vi "Test Error Test.vi"(8 "error in (no error)":errorcluster, 11 "LUnit Test Case V2 Test Double in":refnum<class "LUnit Test Case V2 Test Double.lvclass">) -> (0 "error out":errorcluster, 3 "LUnit Test Case V2 Test Double out":refnum<class "LUnit Test Case V2 Test Double.lvclass">)   [LabVIEW 2020, in "LUnit Test Case V2 Test Double.lvclass"]
uses:
  LUnit Test Case V2 Test Double.lvclass
  C:/Git/astemes-lunit/source/Rewrite Project/LUnit Test Case/LUnit Test Case V2.lvclass
  LUnit Test Case/LUnit Test Case V2.lvclass/LUnit Test Case V2.ctl
  LUnit Test Case/Private/Append Result.vi
  LUnit Test Case/LUnit Test Case V2.lvclass
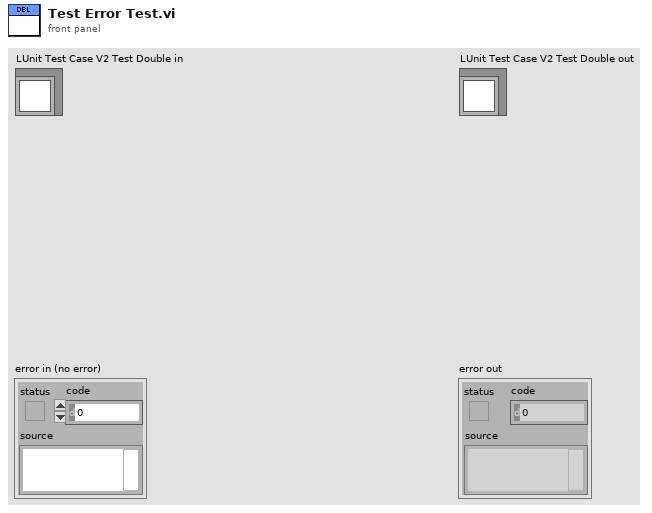
[diagram p1: front panel]
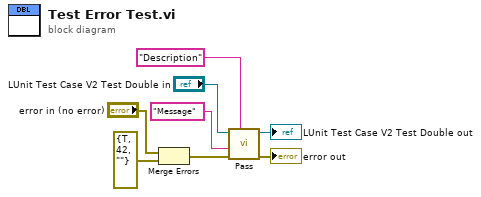
[diagram p0: block diagram]
diagram:
  n1 = Merge Errors("error in (no error)", errorcluster {"status"=TRUE, "code"=42, "source"=""} ("error in (no error)")) -> (w2:errorcluster)
  n2 = call "Pass.vi"("Description"="Description", "error in (no error)"=w2, "Message"="Message", "LUnit Test Case In"="LUnit Test Case V2 Test Double in") -> ("error out"=→"error out":errorcluster, "LUnit Test Case Out"=→"LUnit Test Case V2 Test Double out":refnum<class "LUnit Test Case V2 Test Double.lvclass">)  [unwired: 6 in]
